vi "Request OD Entry Values.vi"(8 "error in":errorcluster, 10 "Index":u16 format="%.0x", 11 "Interactor in":refnum<class "Interactor.lvclass">) -> (0 "error out":errorcluster, 3 "Interactor out":refnum<class "Interactor.lvclass">)   [LabVIEW 2024, in "Interactor.lvlib" / "Interactor.lvclass"]
uses:
  Interactor.lvclass
  Interactor.lvclass/Interactor.ctl
  Object Dictionary UI Messages/Set OD Entry Values Msg/Set OD Entry Values Msg.lvclass/Set OD Entry Values Msg.ctl
  <vilib>/ActorFramework/Message Enqueuer/Message Enqueuer.lvclass/Message Enqueuer.ctl
  Object Dictionary UI Messages/Set OD Entry Values Msg/Set OD Entry Values Msg.lvclass
  C:/Program Files/National Instruments/LabVIEW 2025/vi.lib/ActorFramework/Message/Message.lvclass
  EDS-File-Viewer/source/Electronic Datasheet/Electronic Datasheet.lvclass
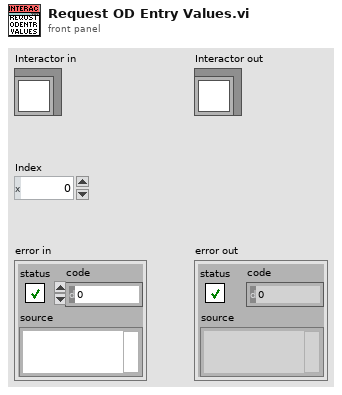
[diagram p1: front panel]
types:
  T1 = cluster{"Multiplexer":cluster{"Index":u16, "Sub-Index":i16}, "Value":u8[]}[][]
  T2 = cluster{"Multiplexer":cluster{"Index":u16, "Sub-Index":i16}, "Value":u8[]}[]
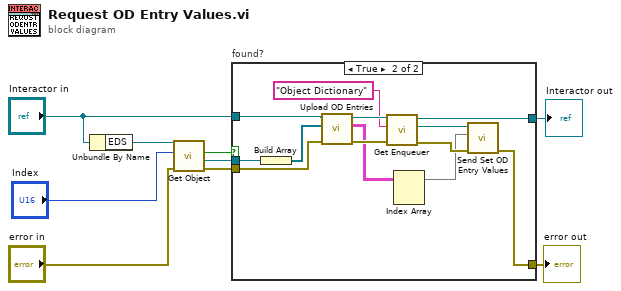
[diagram p0: block diagram]
diagram:
  n1 = Unbundle By Name("Interactor in") -> ("EDS"=w9:refnum<class "Electronic Datasheet.lvclass">)
  n2 = call "Get Object.vi"("error in"="error in", "Index"="Index", "reference in"=w9) -> ("error out"=w4:errorcluster, "OD Entry"=w6:refnum<class "OD Entry.lvclass">, "Found?"=w1:bool)  [unwired: 5 in, 1 out]
  n3 = case "found?" shown="True" w1 {
    tunnel: w6 -> [_ w14]
    tunnel: "Interactor in" -> [w10 w24]
    tunnel: w4 -> [w11 w16]
    tunnel: [w10 w20] -> w3
    tunnel: [w11 w17] -> w2
    frame False {
    }
    frame True {
      n4 = Build Array(w14) -> (w15:refnum<class "OD Entry.lvclass">[])
      n5 = call-dynamic "Upload OD Entries.vi"("error in"=w16, "Entries"=w15, "Interactor in"=w24) -> ("error out"=w21:errorcluster, "Values"=w13:T1, "Interactor out"=w23:refnum<class "Interactor.lvclass">)  [unwired: 6 in]
      n6 = call "Get Enqueuer.vi"("error in"=w21, "Ident"="Object Dictionary", "Interactor in"=w23) -> ("error out"=w18:errorcluster, "Enq"=w19:refnum<class "Message Enqueuer.lvclass">, "Interactor out"=w20:refnum<class "Interactor.lvclass">)  [unwired: 6 in]
      n7 = Index Array(array=w13) -> (element=w12:T2)  [unwired: 2 in]
      n8 = call "Send Set OD Entry Values.vi"("error in (no error)"=w18, "Values"=w12, "Message Enqueuer"=w19) -> ("error out"=w17:errorcluster)  [unwired: 7 in, 1 out]
    }
  }
  "error out" <- w2
  "Interactor out" <- w3
